vi "subtractUnmarkedSum.vi"(10 "Numeric":i32, 11 "BingoBoard in":refnum<class "BingoBoard.lvclass">) -> (3 "output cluster":refnum<class "BingoBoard.lvclass">)   [LabVIEW 2017, in "BingoBoard.lvclass"]
uses:
  BingoBoard.lvclass
  BingoBoard.lvclass/BingoBoard.ctl
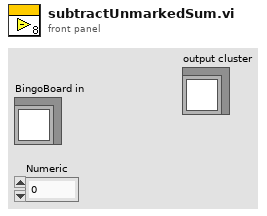
[diagram p1: front panel]
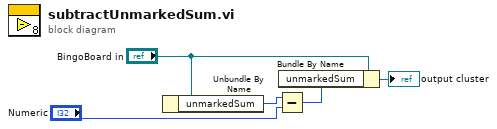
[diagram p0: block diagram]
diagram:
  n1 = Unbundle By Name("BingoBoard in") -> ("unmarkedSum"=w3:i32)
  n2 = Subtract(x=w3, y="Numeric") -> (x-y=w1:i32)
  n3 = Bundle By Name(cluster="BingoBoard in", "unmarkedSum"=w1) -> (→"output cluster":refnum<class "BingoBoard.lvclass">)
